vi "Create Child Actor.vi"(7 "App Inst":refnum<vi>, 8 "error in (no error)":errorcluster, 9 "Actor Name":string, 10 "Parent Class":refnum<vi>, 11 "Library in":refnum<vi>) -> (0 "error out":errorcluster, 3 "Library out":refnum<vi>)   [LabVIEW 2020, in "Add Actor.lvlib"]
uses:
  Add Actor.lvlib
  <vilib>/Utility/EditLVLibs/Edit LVLibs.lvlib
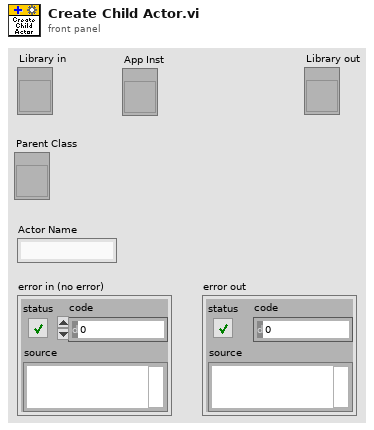
[diagram p1: front panel]
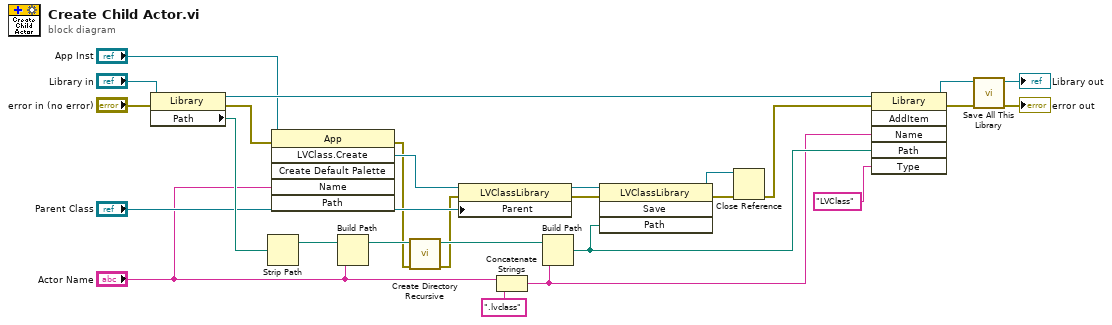
[diagram p0: block diagram]
diagram:
  n1 = property class="Library"(reference="Library in", error in="error in (no error)") -> (reference out=w25:refnum<vi>, error out=w18:errorcluster, "Path"=w22:path)
  n2 = Strip Path(path=w22) -> (stripped path=w12:path)  [unwired: 1 out]
  n3 = invoke class="App" method="LVClass.Create"(reference="App Inst", error in=w18, "Name"="Actor Name") -> (error out=w7:errorcluster, "LVClass.Create"=w17:refnum<vi>)  [unwired: 3 in, 4 out]
  n4 = Build Path(base path=w12, name or relative path="Actor Name") -> (appended path=w9:path)
  n5 = call <vilib>:"Create Directory Recursive.vi"("error in (no error)"=w7, "directory"=w9) -> ("error out"=w6:errorcluster, "directory copy"=w8:path)  [unwired: 3 in, 1 out]
  n6 = property class="LVClassLibrary"(reference=w17, error in=w6, "Parent"="Parent Class") -> (reference out=w23:refnum<vi>, error out=w27:errorcluster)
  n7 = Concatenate Strings("Actor Name", ".lvclass" ("string")) -> (w10:string)
  n8 = Build Path(base path=w8, name or relative path=w10) -> (appended path=w20:path)
  n9 = invoke class="LVClassLibrary" method="Save"(reference=w23, error in=w27, "Path"=w20) -> (reference out=w16:refnum<vi>, error out=w15:errorcluster)  [unwired: 1 in, 2 out]
  n10 = Close Reference(reference=w16, error in (no error)=w15) -> (error out=w13:errorcluster)
  n11 = invoke class="Library" method="AddItem"(reference=w25, error in=w13, "Name"=w10, "Path"=w20, "Type"="LVClass") -> (reference out=w2:refnum<vi>, error out=w4:errorcluster)  [unwired: 1 in, 4 out]
  n12 = call <vilib>:"Save All This Library.vi"("error in (no error)"=w4, "Library in"=w2) -> ("error out"=→"error out":errorcluster, "Library out"=→"Library out":refnum<vi>)  [unwired: 8 in]
